vi "VI-Edit XControl XML.vi"(0 "Path":path=path "C:/Users/hancock/Desktop/Argh/Argh.xctl", 11 "error in (no error)":errorcluster) -> (15 "error out":errorcluster)   [LabVIEW 2015]
uses:
  <vilib>/xml/Load XML File.vi
  <vilib>/xml/Close Reference(Node).vi
  <vilib>/regexp/Match Regular Expression.xnode
  <vilib>/xml/NI_XML.lvlib
  <resource>/objmgr/DOMUserDefRef.rc
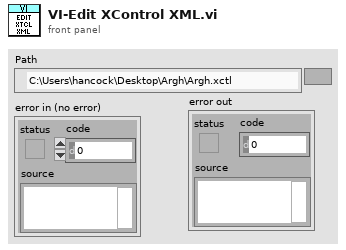
[diagram p1: front panel]
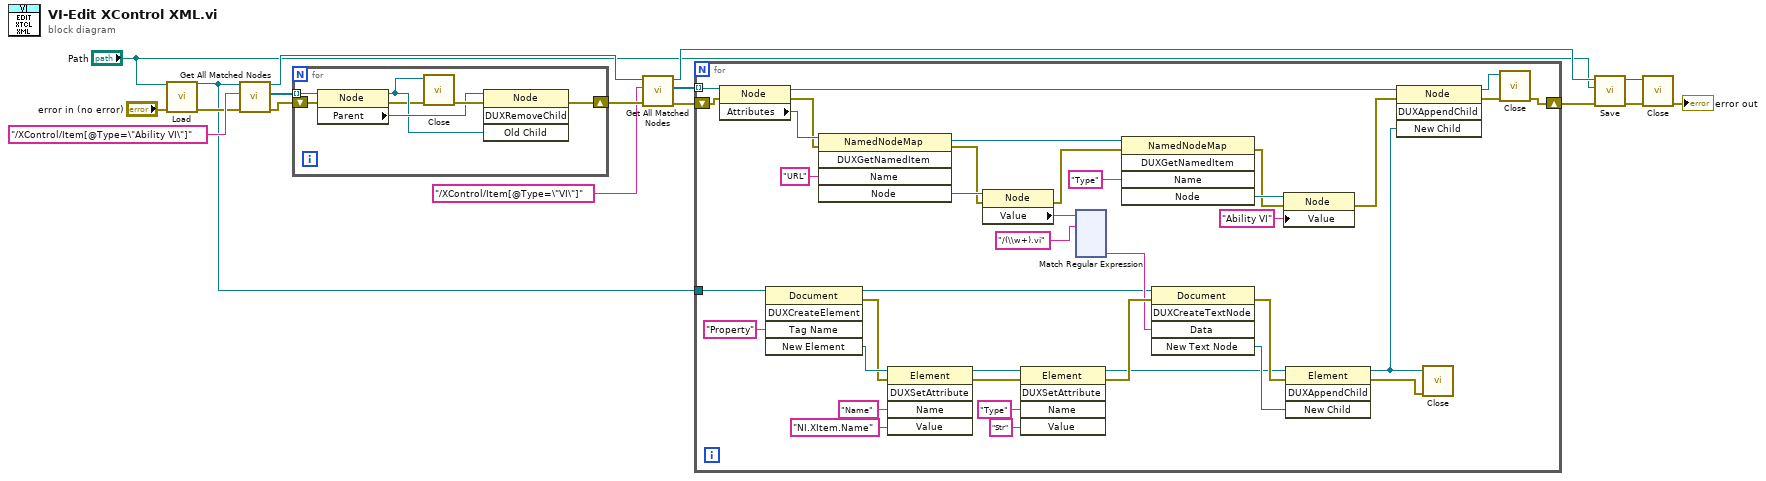
[diagram p0: block diagram]
diagram:
  n1 = call-poly <vilib>:"Load.vi"("path to XML document"="Path", "error in (no error)"="error in (no error)") -> ("DOM document out"=w4:refnum<k20>, "error out"=w14:errorcluster)  [unwired: 11 in, 1 out]
  n2 = call <vilib>:"Get All Matched Nodes.vi"("error in (no error)"=w14, "XPath expression"="/XControl/Item[@Type=\"Ability VI\"]", "node in"=w4) -> ("error out"=w15:errorcluster, "node result array"=w16:refnum<k20>[], "node out"=w10:refnum<k20>)  [unwired: 6 in]
  n3 = for {
    tunnel: w16 -> [w22] mode=indexing
    shift-right: [w23] -> w11
    shift-left: w15 -> [w21]
    n4 = property class="Node"(reference=w22, error in=w21) -> (reference out=w19:refnum<k20>, error out=w18:errorcluster, "Parent"=w20:refnum<k20>)
    n5 = call-poly <vilib>:"Close.vi"("error in (no error)"=w18, "node"=w19) -> ("error out"=w23:errorcluster)  [unwired: 7 out]
    n6 = invoke class="Node" method="DUXRemoveChild"(reference=w20, "Old Child"=w19) -> ()  [unwired: 2 in, 4 out]
  }
  n7 = call <vilib>:"Get All Matched Nodes.vi"("error in (no error)"=w11, "XPath expression"="/XControl/Item[@Type=\"VI\"]", "node in"=w10) -> ("error out"=w6:errorcluster, "node result array"=w8:refnum<k20>[], "node out"=w7:refnum<k20>)  [unwired: 6 in]
  n8 = for {
    tunnel: w8 -> [w61] mode=indexing
    shift-right: [w31] -> w5
    shift-left: w6 -> [w60]
    tunnel: w4 -> [w45]
    n9 = property class="Node"(reference=w61, error in=w60) -> (reference out=w46:refnum<k20>, error out=w53:errorcluster, "Attributes"=w59:refnum<k20>)
    n10 = invoke class="Document" method="DUXCreateElement"(reference=w45, "Tag Name"="Property") -> (reference out=w25:refnum<k20>, error out=w35:errorcluster, "New Element"=w42:refnum<k20>)  [unwired: 3 in, 2 out]
    n11 = invoke class="NamedNodeMap" method="DUXGetNamedItem"(reference=w59, error in=w53, "Name"="URL") -> (reference out=w54:refnum<k20>, error out=w50:errorcluster, "Node"=w57:refnum<k20>)  [unwired: 2 in, 2 out]
    n12 = invoke class="Element" method="DUXSetAttribute"(reference=w42, error in=w35, "Name"="Name", "Value"="NI.XItem.Name") -> (reference out=w37:refnum<k20>, error out=w36:errorcluster)  [unwired: 1 in, 3 out]
    n13 = property class="Node"(reference=w57, error in=w50) -> (error out=w49:errorcluster, "Value"=w56:string)  [unwired: 1 out]
    n14 = invoke class="Element" method="DUXSetAttribute"(reference=w37, error in=w36, "Name"="Type", "Value"="Str") -> (reference out=w24:refnum<k20>, error out=w29:errorcluster)  [unwired: 1 in, 3 out]
    n15 = xnode "Match Regular Expression"("input string"=w56, "regular expression"="/(\\w+).vi") -> ("submatch 1"=w28:string)  [unwired: 4 in, 5 out]
    n16 = invoke class="NamedNodeMap" method="DUXGetNamedItem"(reference=w54, error in=w49, "Name"="Type") -> (error out=w48:errorcluster, "Node"=w51:refnum<k20>)  [unwired: 2 in, 3 out]
    n17 = invoke class="Document" method="DUXCreateTextNode"(reference=w25, error in=w29, "Data"=w28) -> (error out=w27:errorcluster, "New Text Node"=w26:refnum<k20>)  [unwired: 2 in, 3 out]
    n18 = property class="Node"(reference=w51, error in=w48, "Value"="Ability VI" ("Node Value")) -> (error out=w43:errorcluster)  [unwired: 1 out]
    n19 = invoke class="Element" method="DUXAppendChild"(reference=w24, error in=w27, "New Child"=w26) -> (reference out=w34:refnum<k20>, error out=w33:errorcluster)  [unwired: 1 in, 2 out]
    n20 = invoke class="Node" method="DUXAppendChild"(reference=w46, error in=w43, "New Child"=w34) -> (reference out=w30:refnum<k20>, error out=w32:errorcluster)  [unwired: 1 in, 2 out]
    n21 = call-poly <vilib>:"Close.vi"("error in (no error)"=w33, "node"=w34) -> ()  [unwired: 7 in, 1 out]
    n22 = call-poly <vilib>:"Close.vi"("error in (no error)"=w32, "node"=w30) -> ("error out"=w31:errorcluster)  [unwired: 7 in]
  }
  n23 = call <vilib>:"Save.vi"("error in (no error)"=w5, "XML file path"="Path", "DOM document in"=w7) -> ("error out"=w12:errorcluster, "DOM document out"=w13:refnum<k20>)  [unwired: 6 in, 1 out]
  n24 = call-poly <vilib>:"Close.vi"("error in (no error)"=w12, "node"=w13) -> ("error out"=→"error out":errorcluster)  [unwired: 7 out]
